vi "Information.vi"(8 "error in (no error)":errorcluster, 9 "Context":T1, 10 "Information":refnum<class "Information.lvclass">, 11 "Application Controller in":refnum<class "Application Controller.lvclass">) -> (0 "error out":errorcluster, 3 "Application Controller out":refnum<class "Application Controller.lvclass">)   [LabVIEW 2021, in "Application Controller.lvclass"]
uses:
  Application Controller.lvclass
  Publish-Subscribe/Interfaces/Subscriber Messages/Information Msg/Information Msg.lvclass
  Publish-Subscribe/Interfaces/Information/Information.lvclass
  Publish-Subscribe/Context.ctl
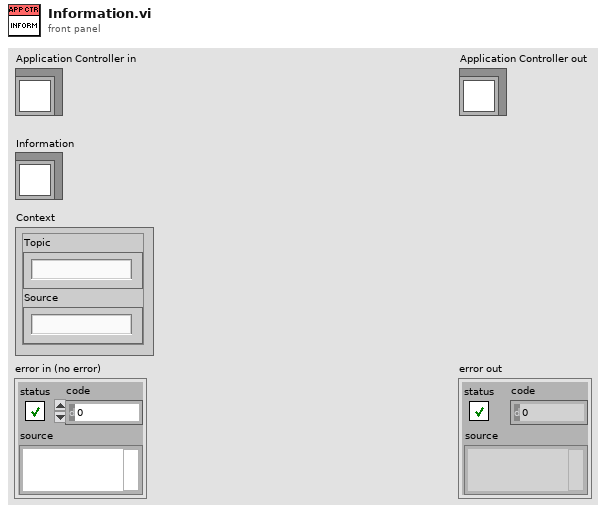
[diagram p1: front panel]
types:
  T1 = typedef "Context.ctl" = cluster{"Topic":string, "Source":string}
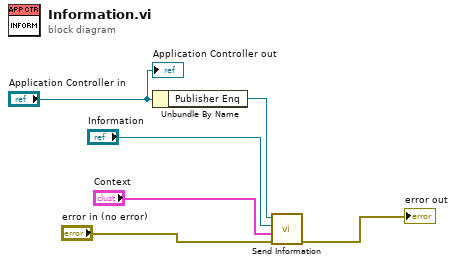
[diagram p0: block diagram]
diagram:
  n1 = Unbundle By Name("Application Controller in") -> ("Publisher Enq"=w6:refnum<class "Message Enqueuer.lvclass">)
  n2 = call "Send Information.vi"("error in (no error)"="error in (no error)", "Context"="Context", "Information"="Information", "Message Enqueuer"=w6) -> ("error out"=→"error out":errorcluster)  [unwired: 6 in, 1 out]
  "Application Controller out" <- "Application Controller in"
